vi "Intacc Controller.vi"(8 "error in":errorcluster) -> ()   [LabVIEW 2019]
doc: "This VI executes continuously carrying out the current operation and responding to updates or new operations. It will often contain the timing or control code that is difficult to place directly in TeleOp. This VI generally opens all sensors and motors and isolates the rest of the robot code from knowing how the operations are carried out."
uses:
  <vilib>/Rock Robotics/WPI/Framework/Completion Status.ctl
  Intacc Setpoints.ctl
  Intacc Operations.ctl
  <vilib>/Rock Robotics/WPI/ThirdParty/REV Robotics/SPARK MAX/Typedef/Spark MAX Control Type.ctl
  Framework/Robot Global Data.vi
  <vilib>/Rock Robotics/Network Tables/NT Write Boolean.vi
panel:
  in  "Interactive Values":T1
  out "Current\nCmd":string
  in  "Buttons":cluster{"Execute Cmd":bool, "Abort Cmd":bool}
  out "Command Timing":cluster{"Start Time (ms)":u32, "Iterations":i32}
  out "Status":T3
  # "Tip: It may be helpful to observe inputs and sensor values.\nYou may also want to display tuning or debugging controls."
  # "Interactive Command: You may fill in the settings for a command\nand schedule it with the Execute button. You can observe and abort\nany command while fine tuning the code for the controller."
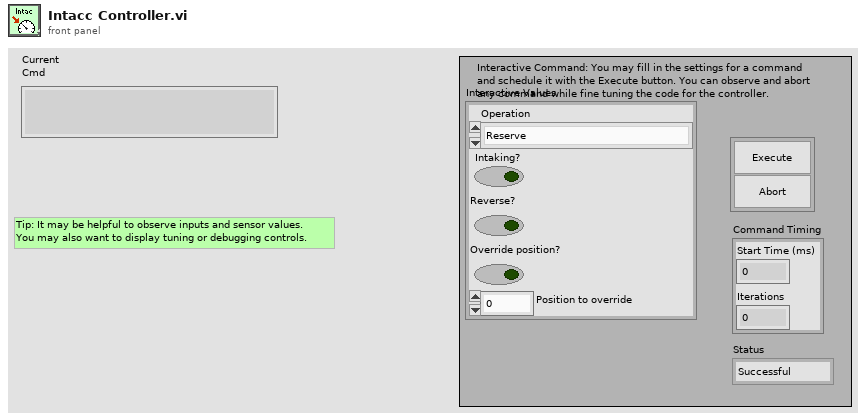
[diagram p1: front panel]
types:
  T1 = typedef "Intacc Setpoints.ctl" = cluster{"Operation":T2, "Intaking?":bool, "Reverse?":bool, "Override position?":bool, "Position to override":dbl}
  T2 = typedef "Intacc Operations.ctl" = enum16{"Reserve", "Read Current", "Immediate"}
  T3 = typedef "Completion Status.ctl" = enum16{"Successful", "Aborted", "Incomplete"}
  T4 = cluster{"P Gain":dbl, "I Gain":dbl, "D Gain":dbl, "F Gain":dbl, "I Zone":dbl, "Min Output":dbl, "Max Output":dbl}
  T5 = typedef "WPI_MotorControlDeviceRef.ctl" = cluster{"DeviceStatus":errorcluster, "Type":T6, "PWM":cluster{"PWM Channel":T7, "DeadBand":T8}, "CAN":cluster{"Device Number":u8, "SetOutput VI Ref":variant, "GetOutput VI Ref":variant, "Enable VI Ref":variant, "Disable VI Ref":variant, "Data":variant}, "Invert":bool, "DIO PWM":cluster{"PWM \"Enable\" Channel":T7, "DIOChannel":T9, "PWM Rate":dbl}}
  T6 = typedef "WPI_MotorControlType.ctl" = enum16{"PWM", "CAN", "DIO PWM"}
  T7 = typedef "FPGA_DIOPWMChannel.ctl" = enum8{"PWM 0", "PWM 1", "PWM 2", "PWM 3", "PWM 4", "PWM 5", "PWM 6", "PWM 7", "PWM 8", "PWM 9", "PWM MXP 0", "PWM MXP 1", "PWM MXP 2", "PWM MXP 3", "PWM MXP 4", "PWM MXP 5", "PWM MXP 6", "PWM MXP 7", "PWM MXP 8", "PWM MXP 9", "Invalid"}
  T8 = typedef "WPI_PWMDeadband.ctl" = cluster{"Name":string, "maxPositivePwm":i32, "minPositivePwm":i32, "centerPwm":i32, "maxNegativePwm":i32, "minNegativePwm":i32, "angularRange":u16}
  T9 = typedef "FPGA_DIOChannel.ctl" = enum8{"DIO 0", "DIO 1", "DIO 2", "DIO 3", "DIO 4", "DIO 5", "DIO 6", "DIO 7", "DIO 8", "DIO 9", "DIO MXP 0", "DIO MXP 1", "DIO MXP 2", "DIO MXP 3", "DIO MXP 4", "DIO MXP 5", "DIO MXP 6", "DIO MXP 7", "DIO MXP 8", "DIO MXP 9", "DIO MXP 10", "DIO MXP 11", "DIO MXP 12", "DIO MXP 13", "DIO MXP 14", "DIO MXP 15", "SPI Port CS1", "SPI Port CS2", "SPI Port CS3", "SPI Port MISO", "SPI Port MOSI", "Invalid"}
  T10 = typedef "Command Status Info.ctl" = cluster{"Name":string, "Status":T3, "notifier out":T11}
  T11 = typedef "Completion Notifier.ctl" = refnum<notifier>
  T12 = cluster{"Current Command":T1, "Command Timing":cluster{"Start Time (ms)":u32, "Iterations":i32}, "Command Arguments":cluster{"Command Info":T10, "Description":string, "Default Command":T1, "queue out":refnum<queue>, "Subsystem Name":string}}
  T13 = typedef "Spark MAX Control Type.ctl" = enum16{"Percent VBus", "Voltage", "Velocity", "Position", "Smart Motion", "Current", "Smart Velocity"}
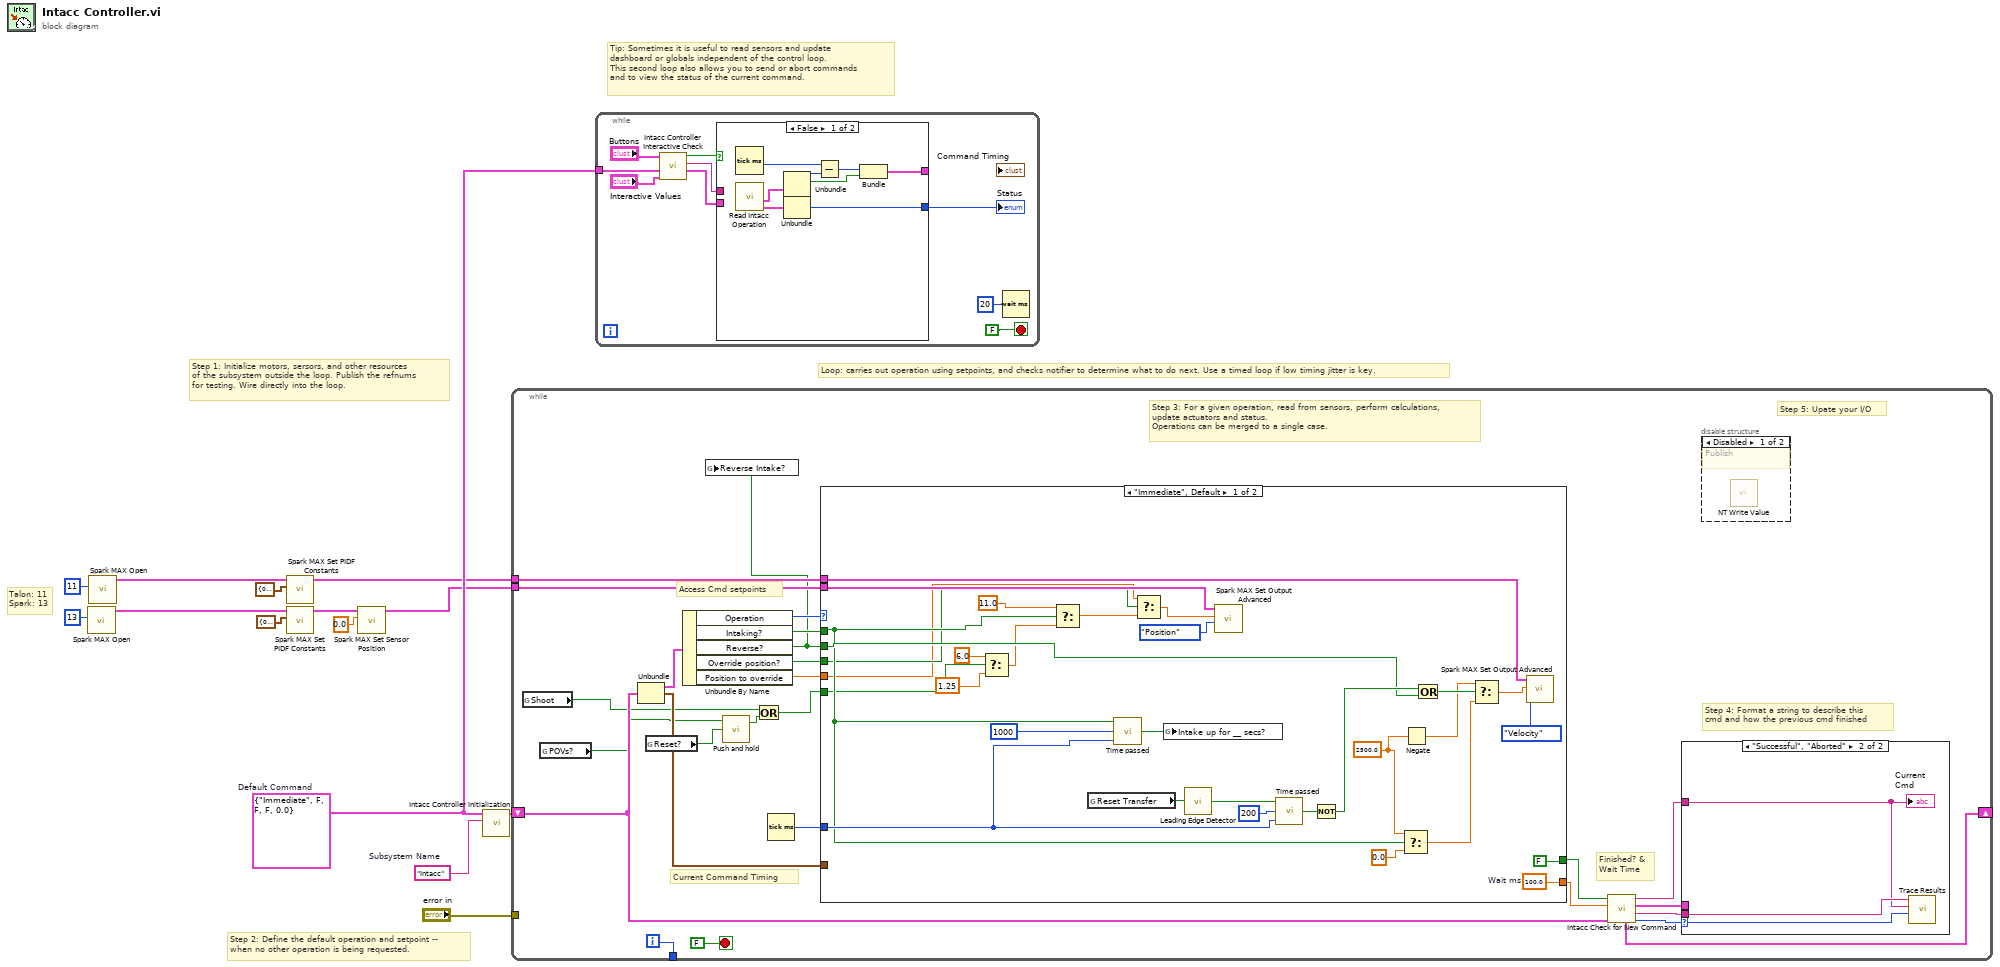
[diagram p0: block diagram]
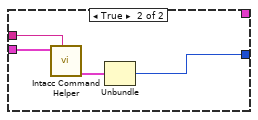
[diagram p2: hidden frame]
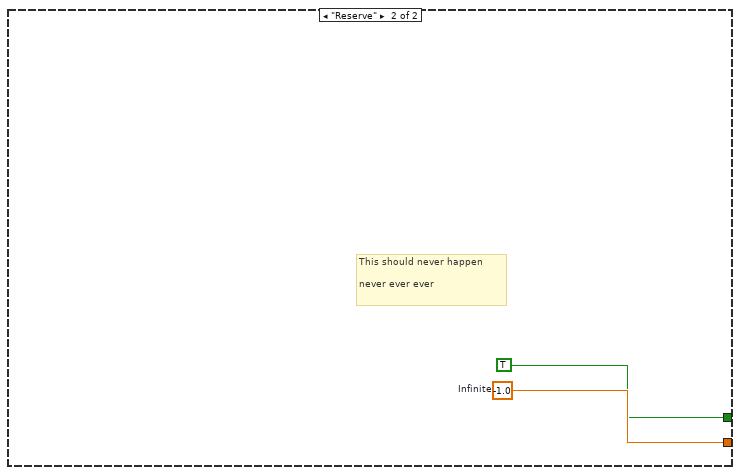
[diagram p5: hidden frame]
diagram:
  w11 = T1 {"Operation"=enum."Immediate", "Intaking?"=FALSE, "Reverse?"=FALSE, "Override position?"=FALSE, "Position to override"=0.0}  # Default Command
  w12 = "Intacc"  # Subsystem Name
  # "Talon: 11\nSpark: 13"
  # "Tip: Sometimes it is useful to read sensors and update\ndashboard or globals independent of the control loop.\nThis second loop also allows you to send or abort commands\nand to view the status of the current command."
  # "Step 2: Define the default operation and setpoint --\nwhen no other operation is being requested."
  # "Step 1: Initialize motors, sersors, and other resources\nof the subsystem outside the loop. Publish the refnums\nfor testing. Wire directly into the loop."
  # "Loop: carries out operation using setpoints, and checks notifier to determine what to do next. Use a timed loop if low timing jitter is key."
  n1 = call <vilib>:"Spark MAX Open.vi"("Device Number"=u8 13) -> ("MotorControlDeviceRef"=w9:T5)  [unwired: 9 in, 1 out]
  n2 = call <vilib>:"Spark MAX Open.vi"("Device Number"=u8 11) -> ("MotorControlDeviceRef"=w3:T5)  [unwired: 9 in, 1 out]
  n3 = call <vilib>:"Spark MAX Set PIDF Constants.vi"("PID Constants"=T4 {"P Gain"=0.0003, "I Gain"=0.0, "D Gain"=0.0, "F Gain"=0.0002, "I Zone"=0.0, "Min Output"=-1.0, "Max Output"=1.0}, "MotorControlDeviceRef"=w3) -> ("MotorControlDeviceRef"=w2:T5)  [unwired: 8 in, 1 out]
  n4 = call <vilib>:"Spark MAX Set PIDF Constants.vi"("PID Constants"=T4 {"P Gain"=0.07, "I Gain"=0.0001, "D Gain"=0.0, "F Gain"=0.0, "I Zone"=1.0, "Min Output"=-0.5, "Max Output"=0.5}, "MotorControlDeviceRef"=w9) -> ("MotorControlDeviceRef"=w8:T5)  [unwired: 8 in, 1 out]
  n5 = call <vilib>:"Spark MAX Set Sensor Position.vi"("Position"=0.0, "MotorControlDeviceRef"=w8) -> ("MotorControlDeviceRef"=w7:T5)  [unwired: 8 in, 1 out]
  n6 = call "Intacc Controller Initialization.vi"("Subsystem Name"=w12, "Default Command"=w11) -> ("Current Command"=w13:T12)  [unwired: 9 in]
  n7 = while {
    shift-right: [w33] -> _
    shift-left: w13 -> [w26]
    tunnel: [w38] -> _
    tunnel: "error in" -> [_]
    tunnel: w7 -> [w18]
    tunnel: w2 -> [w25]
    i -> [w38]
    stop <- FALSE stop-if-true
    # "Step 5: Upate your I/O"
    # "Step 4: Format a string to describe this\ncmd and how the previous cmd finished"
    # "Current Command Timing"
    # "Access Cmd setpoints"
    # "Finished? &\nWait Time"
    # "Step 3: For a given operation, read from sensors, perform calculations,\nupdate actuators and status.\nOperations can be merged to a single case."
    n8 = global read "Robot Global Data.vi" "Shoot"() -> (w22:bool)
    n9 = global read "Robot Global Data.vi" "POVs?"() -> (w23:bool)
    n10 = Unbundle(w26) -> ("Current Command"=w37:T1, "Command Timing"=w34:cluster{"Start Time (ms)":u32, "Iterations":i32})  [unwired: 1 out]
    n11 = global read "Robot Global Data.vi" "Reset?"() -> (w24:bool)
    n12 = Unbundle By Name(w37) -> ("Operation"=w36:T2, "Intaking?"=w20:bool, "Reverse?"=w15:bool, "Override position?"=w17:bool, "Position to override"=w16:dbl)
    n13 = global write "Robot Global Data.vi" "Reverse Intake?"(w15) -> ()
    n14 = call "Push and hold.vi"("Reset"=w24, "Input"=w23) -> ("Output"=w21:bool)  [unwired: 2 in]
    n15 = Or(x=w22, y=w21) -> (x .or. y?=w19:bool)
    n16 = Tick Count (ms)() -> (millisecond timer value=w35:u32)
    n17 = case shown="\"Immediate\", Default" w36 {
      tunnel: [w73 w75] -> w31
      tunnel: [FALSE ("ignore previous (F)") TRUE ("ignore previous (F)")] -> w32
      tunnel: w34 -> [_ _]
      tunnel: w20 -> [w55 _]
      tunnel: w35 -> [w67 _]
      tunnel: w18 -> [w62 _]
      tunnel: w25 -> [w49 _]
      tunnel: w19 -> [w46 _]
      tunnel: w15 -> [w56 _]
      tunnel: w17 -> [w51 _]
      tunnel: w16 -> [w50 _]
      frame "Immediate", Default {
        w43 = 2500.0 ("Intake Vel")
        w73 = 100.0  # Wait ms
        n18 = Select(t=6.0, s=w46, f=1.25 ("5")) -> (s? t:f=w54:dbl)
        n19 = Select(t=11.0 ("20"), s=w55, f=w54) -> (s? t:f=w53:dbl)
        n20 = global read "Robot Global Data.vi" "Reset Transfer"() -> (w64:bool)
        n21 = call "Time passed.vi"("ms timer value"=w67, "Wait time"=u32 1000, "Reset"=w55) -> ("Boolean out"=w68:bool)
        n22 = Select(t=w50, s=w51, f=w53) -> (s? t:f=w52:dbl)
        n23 = global write "Robot Global Data.vi" "Intake up for __ secs?"(w68) -> ()
        n24 = call "Leading Edge Detector.vi"("Boolean"=w64) -> ("Out"=w63:bool)
        n25 = call <vilib>:"Spark MAX Set Output Advanced.vi"("Control Mode"=Spark_MAX_Control_Type."Position", "Setpoint"=w52, "MotorControlDevRef"=w62) -> ()  [unwired: 7 in, 2 out]
        n26 = call "Time passed.vi"("ms timer value"=w67, "Wait time"=u32 200, "Reset"=w63) -> ("Boolean out"=w65:bool)
        n27 = Not(x=w65) -> (.not. x?=w58:bool)
        n28 = Select(t=w43, s=w55, f=0.0) -> (s? t:f=w45:dbl)
        n29 = Negate(x=w43) -> (-x=w44:dbl)
        n30 = Or(x=w58, y=w56) -> (x .or. y?=w57:bool)
        n31 = Select(t=w44, s=w57, f=w45) -> (s? t:f=w47:dbl)
        n32 = call <vilib>:"Spark MAX Set Output Advanced.vi"("Control Mode"=Spark_MAX_Control_Type."Velocity", "Setpoint"=w47, "MotorControlDevRef"=w49) -> ()  [unwired: 7 in, 2 out]
      }
      frame "Reserve" {
        w75 = -1.0  # Infinite
        # "This should never happen\n\nnever ever ever"
      }
    }
    n33 = call "Intacc Check for New Command.vi"("Current Command"=w26, "Wait time (ms)"=w31, "Finished?"=w32) -> ("Completion"=w27:T3, "Subsystem Name"=w28:string, "Current Command"=w29:T1, "Initial Trace String"=w30:string, "NextCommand"=w33:T12)  [unwired: 4 in]
    n34 = case shown="\"Successful\", \"Aborted\"" w27 {
      selector: w27 -> [_ w42]
      tunnel: w30 -> [_ w40]
      tunnel: w29 -> [_ _]
      tunnel: w28 -> [_ w41]
      frame "Incomplete", Default {
        # "Continuing current command"
      }
      frame "Successful", "Aborted" {
        # "Report and setup for next command"
        n35 = call <vilib>:"Trace Results.vi"("Status of previous command"=w42, "Description"=w40, "Subsystem"=w41) -> ()  [unwired: 9 in]
        "Current\nCmd" <- w40
      }
    }
    n36 = disable-structure shown="Disabled" {
      frame Disabled {
        # "Publish"
        n37 = call-poly <vilib>:"NT Write Value.vi"() -> ()  [unwired: 11 in, 1 out]
      }
      frame Enabled {
      }
    }
  }
  n38 = while {
    tunnel: w11 -> [w81]
    stop <- FALSE stop-if-true
    n39 = call "Intacc Controller Interactive Check.vi"("Interactive Command in"="Interactive Values", "Default Command"=w81, "Buttons"="Buttons") -> ("Interactive Command out"=w78:T1, "Trace String"=w79:string, "Schedule"=w80:bool)  [unwired: 6 in]
    n40 = case shown="False" w80 {
      tunnel: [w92 w96] -> w77
      tunnel: w78 -> [_ w94]
      tunnel: [w88 _] -> _
      tunnel: w79 -> [_ w95]
      frame False {
        n41 = Tick Count (ms)() -> (millisecond timer value=w87:u32)
        n42 = call "Read Intacc Operation.vi"() -> ("Command Info"=w85:T10, "SubSystem Data"=w86:T1)  [unwired: 9 in, 1 out]
        n43 = Unbundle(w86) -> ("Operation"=w91:T2, "Intaking?"=w89:bool)  [unwired: 3 out]
        n44 = Unbundle(w85) -> ("Status"=w92:T3)  [unwired: 2 out]
        n45 = Subtract(x=w87, y=w91) -> (x-y=w90:u32)
        n46 = Bundle(w90, "Intaking?"=w89) -> (w88:cluster{u32, "Intaking?":bool})  [unwired: 1 in]
      }
      frame True {
        n47 = call "Intacc Command Helper.vi"("Description"=w95, "SubSystem Data"=w94) -> ("Command Info Out"=w93:T10)  [unwired: 7 in, 2 out]
        n48 = Unbundle(w93) -> ("Status"=w96:T3)  [unwired: 2 out]
      }
    }
    "Status" <- w77
    n49 = Wait (ms)(milliseconds to wait=u32 20) -> ()  [unwired: 1 out]
  }
